vi "Q-Create.vi"(7 "max queue size (-1, unlimited)":i32=1, 8 "error in":errorcluster, 10 "Queue Type":T1, 11 "Q Name":string) -> (0 "error out":errorcluster)   [LabVIEW 2016]
uses:
  PSDAQEG_Task Queue Type.ctl
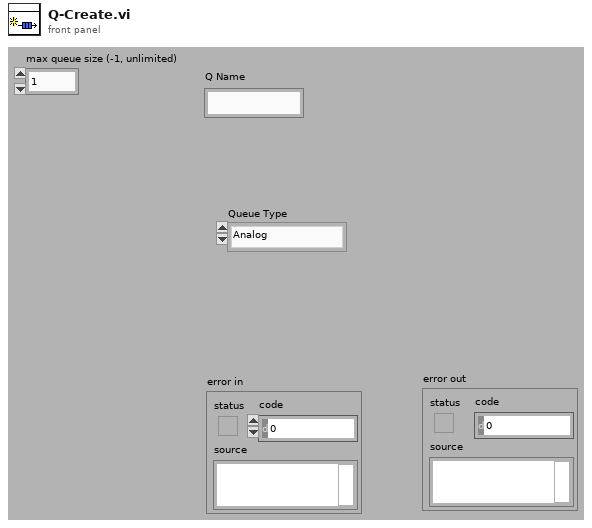
[diagram p1: front panel]
types:
  T1 = typedef "PSDAQEG_Task Queue Type.ctl" = enum16{"Analog", "Digital", "Variant"}
  T2 = cluster{"Analog Data":waveform(dbl)[], "Digital Data":digitalwaveform[], "Variant Data":variant[]}
  T3 = cluster{"max queue size (-1, unlimited)":i32, "Analog Data":waveform(dbl)[]}
  T4 = cluster{"max queue size (-1, unlimited)":i32, "Digital Data":digitalwaveform[]}
  T5 = cluster{"max queue size (-1, unlimited)":i32, "Variant Data":variant[]}
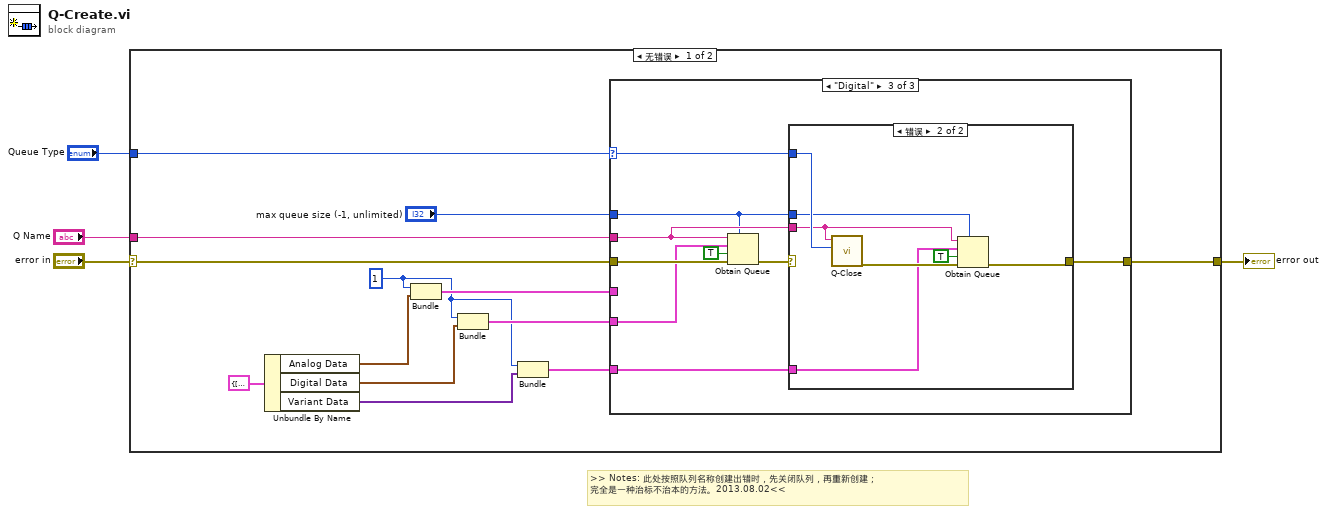
[diagram p0: block diagram]
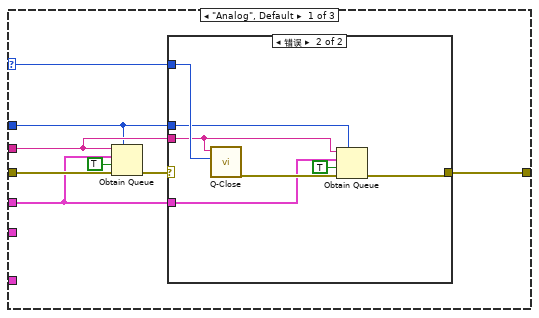
[diagram p2: hidden frame]
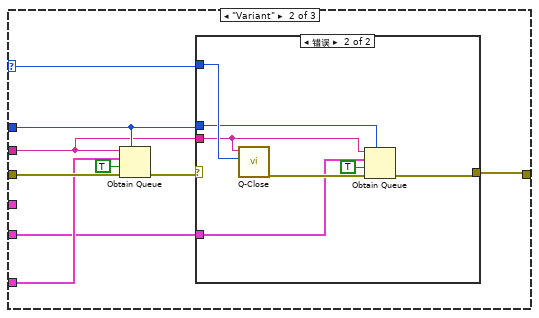
[diagram p4: hidden frame]
diagram:
  # ">> Notes: 此处按照队列名称创建出错时，先关闭队列，再重新创建；\n完全是一种治标不治本的方法。2013.08.02<<"
  n1 = case shown="无错误" "error in" {
    selector: "error in" -> [w6 w68]
    tunnel: "Q Name" -> [w17 _]
    tunnel: "Queue Type" -> [w16 _]
    tunnel: [w14 w68] -> w2
    frame No Error {
      w12 = 1 ("max queue size (-1, unlimited)")
      n2 = Unbundle By Name(T2 {"Analog Data"=[], "Digital Data"=[], "Variant Data"=[]} ("Read Data")) -> ("Analog Data"=w9:waveform(dbl)[], "Digital Data"=w8:digitalwaveform[], "Variant Data"=w7:variant[])
      n3 = Bundle("max queue size (-1, unlimited)"=w12, "Analog Data"=w9) -> (w13:T3)  [unwired: 1 in]
      n4 = Bundle("max queue size (-1, unlimited)"=w12, "Digital Data"=w8) -> (w15:T4)  [unwired: 1 in]
      n5 = Bundle("max queue size (-1, unlimited)"=w12, "Variant Data"=w7) -> (w11:T5)  [unwired: 1 in]
      n6 = case shown="\"Digital\"" w16 {
        selector: w16 -> [w19 w37 w52]
        tunnel: w17 -> [w21 w36 w54]
        tunnel: w6 -> [w25 w42 w59]
        tunnel: "max queue size (-1, unlimited)" -> [w20 w38 w53]
        tunnel: w15 -> [_ w34 w58]
        tunnel: [w22 w35 w55] -> w14
        tunnel: w13 -> [w18 _ _]
        tunnel: w11 -> [_ w41 w51]
        frame "Analog", Default {
          n7 = Obtain Queue(max queue size (-1, unlimited)=w20, name (unnamed)=w21, element data type=w18, create if not found? (T)=TRUE, error in (no error)=w25) -> (error out=w23:errorcluster)  [unwired: 2 out]
          n8 = case shown="错误" w23 {
            selector: w23 -> [w26 _]
            tunnel: [w26 w27] -> w22
            tunnel: w21 -> [_ w29]
            tunnel: w20 -> [_ w28]
            tunnel: w19 -> [_ w33]
            tunnel: w18 -> [_ w30]
            frame No Error {
            }
            frame Error {
              n9 = call "Q-Close.vi"("Queue Type"=w33, "Q Name"=w29) -> ("error out"=w31:errorcluster)  [unwired: 9 in]
              n10 = Obtain Queue(max queue size (-1, unlimited)=w28, name (unnamed)=w29, element data type=w30, create if not found? (T)=TRUE, error in (no error)=w31) -> (error out=w27:errorcluster)  [unwired: 2 out]
            }
          }
        }
        frame "Variant" {
          n11 = Obtain Queue(max queue size (-1, unlimited)=w38, name (unnamed)=w36, element data type=w41, create if not found? (T)=TRUE, error in (no error)=w42) -> (error out=w39:errorcluster)  [unwired: 2 out]
          n12 = case shown="错误" w39 {
            selector: w39 -> [w43 _]
            tunnel: [w43 w44] -> w35
            tunnel: w36 -> [_ w46]
            tunnel: w38 -> [_ w45]
            tunnel: w37 -> [_ w50]
            tunnel: w34 -> [_ w47]
            frame No Error {
            }
            frame Error {
              n13 = call "Q-Close.vi"("Queue Type"=w50, "Q Name"=w46) -> ("error out"=w48:errorcluster)  [unwired: 9 in]
              n14 = Obtain Queue(max queue size (-1, unlimited)=w45, name (unnamed)=w46, element data type=w47, create if not found? (T)=TRUE, error in (no error)=w48) -> (error out=w44:errorcluster)  [unwired: 2 out]
            }
          }
        }
        frame "Digital" {
          n15 = Obtain Queue(max queue size (-1, unlimited)=w53, name (unnamed)=w54, element data type=w58, create if not found? (T)=TRUE, error in (no error)=w59) -> (error out=w56:errorcluster)  [unwired: 2 out]
          n16 = case shown="错误" w56 {
            selector: w56 -> [w60 _]
            tunnel: [w60 w61] -> w55
            tunnel: w54 -> [_ w63]
            tunnel: w53 -> [_ w62]
            tunnel: w52 -> [_ w67]
            tunnel: w51 -> [_ w64]
            frame No Error {
            }
            frame Error {
              n17 = call "Q-Close.vi"("Queue Type"=w67, "Q Name"=w63) -> ("error out"=w65:errorcluster)  [unwired: 9 in]
              n18 = Obtain Queue(max queue size (-1, unlimited)=w62, name (unnamed)=w63, element data type=w64, create if not found? (T)=TRUE, error in (no error)=w65) -> (error out=w61:errorcluster)  [unwired: 2 out]
            }
          }
        }
      }
    }
    frame Error {
    }
  }
  "error out" <- w2
